vi "QueryMirror.vi"(8 "error in (no error)":errorcluster, 10 "Mirror":T1, 11 "DongWoo in":refnum<class "DongWoo.lvclass">) -> (0 "error out":errorcluster, 3 "DongWoo out":refnum<class "DongWoo.lvclass">)   [LabVIEW 2023, in "DongWoo_Spectrometer.lvlib" / "DongWoo.lvclass"]
uses:
  typedefs/SpectroMirrorCtrl.ctl
  DongWoo.lvclass
  DongWoo.lvclass/DongWoo.ctl
  typedefs/typedefs.lvlib
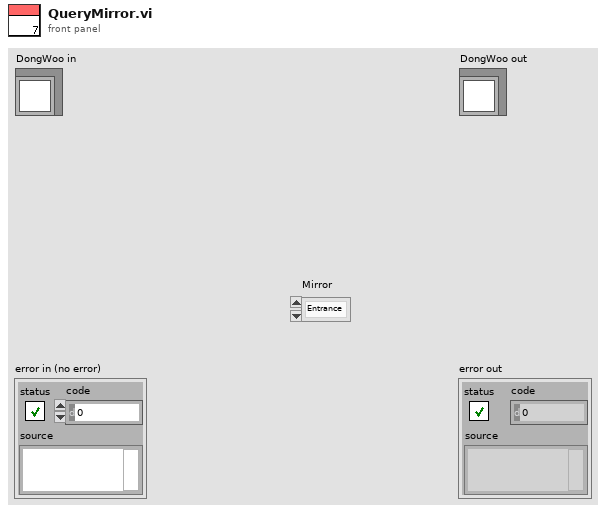
[diagram p1: front panel]
types:
  T1 = typedef "typedefs.lvlib/SpectroMirrorCtrl.ctl" = enum16{"Entrance", "Exit"}
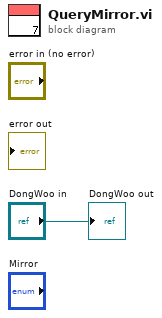
[diagram p0: block diagram]
diagram:
  "DongWoo out" <- "DongWoo in"
